vi "Read Temperature DBL.vi"(8 "error in":errorcluster, 10 "Source":string, 11 "IRead Temperature in":refnum<class "IRead Temperature.lvclass">) -> (0 "error out":errorcluster, 1 "Time Stamp":timestamp format="%<%x %.3X>T", 2 "Temperature":dbl, 3 "IRead Temperature out":refnum<class "IRead Temperature.lvclass">)   [LabVIEW 2024, in "IRead Temperature.lvclass"]
uses:
  IRead Temperature.lvclass
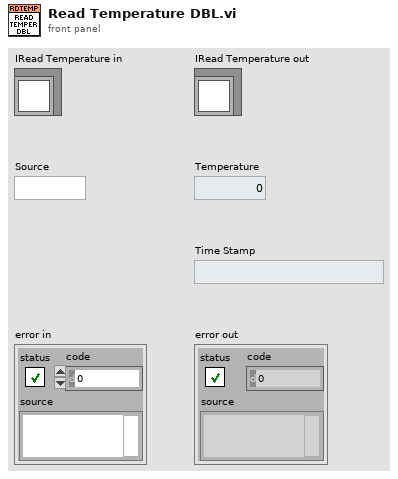
[diagram p1: front panel]
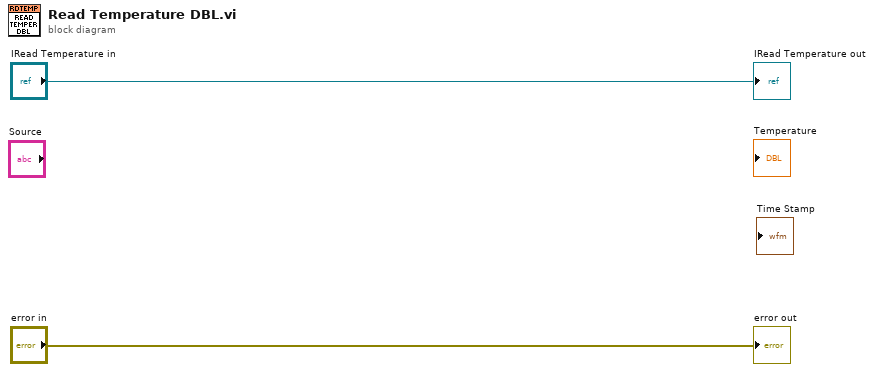
[diagram p0: block diagram]
diagram:
  "error out" <- "error in"
  "IRead Temperature out" <- "IRead Temperature in"
